vi "DataFrom_ini (SubVI).vi"(8 "error in (no error)":errorcluster, 10 "UUT":string, 11 "appended path":path) -> (0 "error out":errorcluster, 1 "FileName":string, 2 "Next SN":i32, 3 "UUT SoftwareVer":string, 4 "ParamVersion":string, 5 "PN":string)   [LabVIEW 2017]
uses:
  <vilib>/Utility/config.llb/Read Key (String).vi
  <vilib>/Utility/config.llb/NI_LVConfig.lvlib
panel:
  out "found?":bool
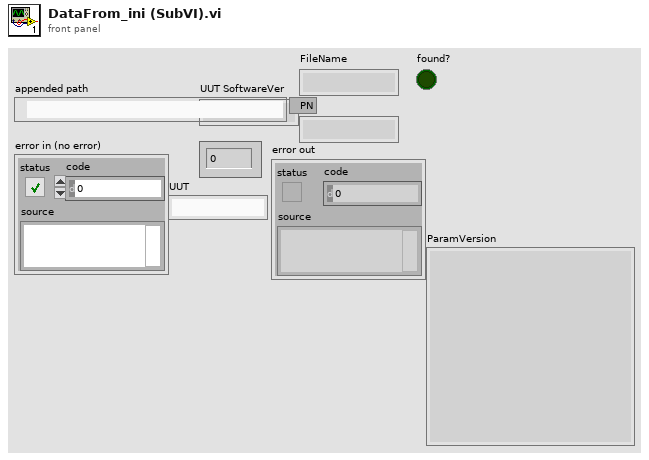
[diagram p1: front panel]
types:
  T1 = typedef "NI_LVConfig.lvlib/Config Data RefNum.ctl" = refnum<k1>
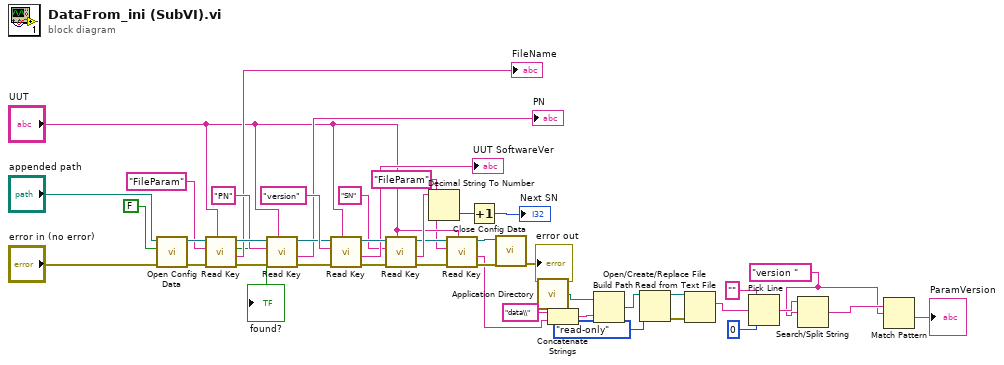
[diagram p0: block diagram]
diagram:
  w3 = "version " ("search string/char (-)")
  n1 = call <vilib>:"Open Config Data.vi"("error in (no error)"="error in (no error)", "create file if necessary (T)"=FALSE, "configuration file path"="appended path") -> ("error out"=w28:errorcluster, "refnum"=w33:T1)  [unwired: 7 out]
  n2 = call-poly <vilib>:"Read Key.vi"("section"="UUT", "error in (no error)"=w28, "key"="FileParam", "refnum"=w33) -> ("error out"=w29:errorcluster, "value"=→"FileName":string, "found?"=→"found?":bool, "refnum out"=w32:T1)  [unwired: 2 in, 2 out]
  n3 = call-poly <vilib>:"Read Key.vi"("section"="UUT", "error in (no error)"=w29, "key"="PN", "refnum"=w32) -> ("error out"=w30:errorcluster, "value"=→"PN":string, "refnum out"=w31:T1)  [unwired: 2 in, 3 out]
  n4 = call-poly <vilib>:"Read Key.vi"("section"="UUT", "error in (no error)"=w30, "key"="version", "refnum"=w31) -> ("error out"=w37:errorcluster, "value"=→"UUT SoftwareVer":string, "refnum out"=w38:T1)  [unwired: 2 in, 3 out]
  n5 = call-poly <vilib>:"Read Key.vi"("section"="UUT", "error in (no error)"=w37, "key"="SN", "refnum"=w38) -> ("error out"=w21:errorcluster, "value"=w42:string, "refnum out"=w20:T1)  [unwired: 2 in, 3 out]
  n6 = Decimal String To Number(string=w42) -> (number=w44:i32)  [unwired: 2 in, 1 out]
  n7 = call-poly <vilib>:"Read Key.vi"("section"="UUT", "error in (no error)"=w21, "key"="FileParam", "refnum"=w20) -> ("error out"=w18:errorcluster, "value"=w12:string, "refnum out"=w19:T1)  [unwired: 2 in, 3 out]
  n8 = Increment(x=w44) -> (x+1=→"Next SN":i32)
  n9 = call <vilib>:"Close Config Data.vi"("error in (no error)"=w18, "refnum"=w19) -> ("error out"=→"error out":errorcluster)  [unwired: 8 in, 1 out]
  n10 = call <vilib>:"Application Directory.vi"() -> ("Application Directory"=w15:path)
  n11 = Concatenate Strings("data\\" ("string"), w12) -> (w14:string)
  n12 = Build Path(base path=w15, name or relative path=w14) -> (appended path=w11:path)
  n13 = Open/Create/Replace File(file path (use dialog)=w11, access (0:read/write)=enum16{"read/write", "read-only", "write-only"}."read-only") -> (refnum out=w8:refnum<file>, error out=w9:errorcluster)  [unwired: 4 in, 1 out]
  n14 = Read from Text File(file (use dialog)=w8, error in=w9) -> (text=w1:string)  [unwired: 2 in, 3 out]
  n15 = Pick Line(string ("")="", multi-line string=w1, line index=0) -> (output string=w5:string)
  n16 = Search/Split String(string=w5, search string/char (-)=w3) -> (match + rest of string=w4:string)  [unwired: 1 in, 2 out]
  n17 = Match Pattern(string=w4, regular expression=w3) -> (after substring=→"ParamVersion":string)  [unwired: 1 in, 3 out]
